vi "Create New Member.vi"(6 "Dynamic?":bool, 8 "Parent":refnum<vi>, 9 "Name":string, 10 "Template":refnum<vi>, 11 "LVClassLibrary":refnum<vi>) -> (2 "Member Item":refnum<vi>, 3 "Member VI":refnum<vi>)   [LabVIEW 2018, in "LVClassByRef.lvlib"]
uses:
  <resource>/Framework/Providers/LVClassByRef/LVClassByRef.lvlib
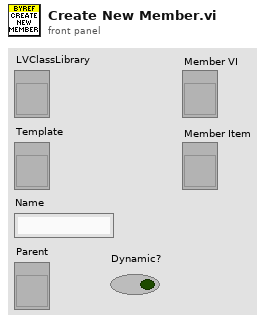
[diagram p1: front panel]
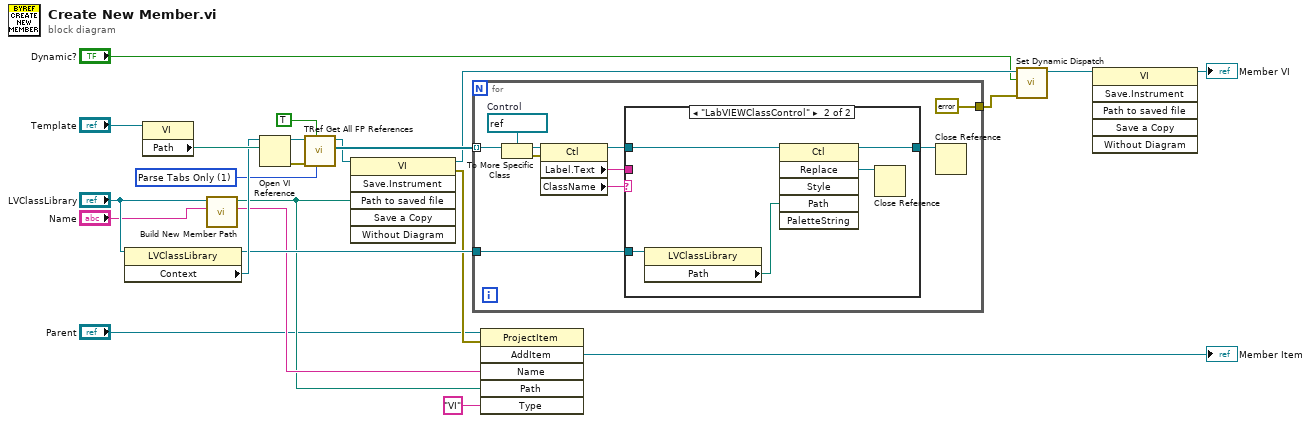
[diagram p0: block diagram]
diagram:
  w19 = u16 1 items=["Parse All", "Parse Tabs Only"] ("Parsing Rule")
  n1 = property class="LVClassLibrary"(reference="LVClassLibrary") -> (reference out=w16:refnum<vi>, "Context"=w22:refnum<vi>)  [unwired: 1 in, 1 out]
  n2 = property class="VI"(reference="Template") -> ("Path"=w23:path)  [unwired: 1 in, 2 out]
  n3 = call <resource>:"Build New Member Path.vi"("Member Name"="Name", "Class"="LVClassLibrary") -> ("New Member Name"=w12:string, "New Member Path"=w11:path)  [unwired: 8 in]
  n4 = Open VI Reference(application reference (local)=w22, vi path=w23) -> (vi reference=w21:refnum<vi>, error out=w18:errorcluster)  [unwired: 4 in]
  n5 = call <vilib>:"TRef Get All FP References.vi"("Parsing Rule"=w19, "Ignore Decorations?"=TRUE, "error in (no error)"=w18, "VI Refnum"=w21) -> ("All FP Objects"=w17:refnum<vi>[], "dup VI Refnum"=w14:refnum<vi>)  [unwired: 3 in, 3 out]
  n6 = invoke class="VI" method="Save.Instrument"(reference=w14, "Path to saved file"=w11) -> (reference out=w3:refnum<vi>, error out=w13:errorcluster)  [unwired: 4 in, 4 out]
  n7 = for {
    tunnel: w17 -> [w32] mode=indexing
    tunnel: w16 -> [w26]
    tunnel: [errorcluster {"status"=FALSE, "code"=0, "source"=""} ("error constant")] -> w1
    w33 = refnum<vi> refnum  # Control
    n8 = To More Specific Class(target class=w33, reference=w32) -> (specific class reference=w31:refnum<vi>, error out=w30:errorcluster)  [unwired: 1 in]
    n9 = property class="Ctl"(reference=w31, error in=w30) -> (reference out=w27:refnum<vi>, "Label.Text"=w28:string, "ClassName"=w29:string)  [unwired: 1 out]
    n10 = case shown="\"LabVIEWClassControl\"" w29 {
      tunnel: w28 -> [_ _]
      tunnel: w27 -> [w34 w39]
      tunnel: w26 -> [_ w38]
      tunnel: [w34 w35] -> w24
      frame Default {
      }
      frame "LabVIEWClassControl" {
        n11 = property class="LVClassLibrary"(reference=w38) -> ("Path"=w37:path)  [unwired: 1 in, 2 out]
        n12 = invoke class="Ctl" method="Replace"(reference=w39, "Path"=w37) -> (reference out=w35:refnum<vi>, "Replace"=w36:refnum<vi>)  [unwired: 4 in, 4 out]
        n13 = Close Reference(reference=w36) -> ()  [unwired: 1 in, 1 out]
      }
    }
    n14 = Close Reference(reference=w24) -> ()  [unwired: 1 in, 1 out]
  }
  n15 = invoke class="ProjectItem" method="AddItem"(reference="Parent", error in=w13, "Name"=w12, "Path"=w11, "Type"="VI") -> ("AddItem"=→"Member Item":refnum<vi>)  [unwired: 1 in, 5 out]
  n16 = call <resource>:"Set Dynamic Dispatch.vi"("error in (no error)"=w1, "Dynamic?"="Dynamic?", "VI Refnum In"=w3) -> ("VI Refnum"=w4:refnum<vi>)  [unwired: 7 in, 1 out]
  n17 = invoke class="VI" method="Save.Instrument"(reference=w4) -> (reference out=→"Member VI":refnum<vi>)  [unwired: 5 in, 5 out]
